vi "mxwScript_API_Option_TemplateRef.vi"(6 "terminalData":T2, 7 "templateRefType":T3, 8 "error in (no error)":errorcluster, 11 "options in":T4[](array[typedef])) -> (0 "error out":errorcluster, 3 "options out":T4[](array[typedef]))   [LabVIEW 2020]
doc: "Sets the default relationship between the template and block diagram reference points. This is used to calculate the drop position of templates."
uses:
  codeGenAPISupport.llb/cgAPI_mxwScript_OptionData.ctl
  codeGenAPISupport.llb/cgAPI_mxwScript_DrpTmplt_TemplateRefType.ctl
  codeGenAPISupport.llb/cgAPI_mxwScript_DrpTmplt_TerminalData.ctl
  codeGenAPISupport.llb/cgAPI_mxwScript_DrpTmplt_ReferencePosition.ctl
panel:
  in  "referencePosition":T1
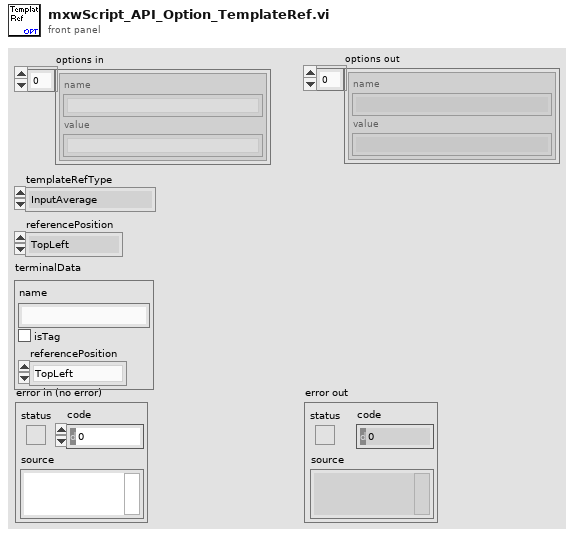
[diagram p1: front panel]
types:
  T1 = typedef "cgAPI_mxwScript_DrpTmplt_ReferencePosition.ctl" = enum16{"TopLeft", "Top", "TopRight", "Left", "Middle", "Right", "BottomLeft", "Bottom", "BottomRight"}
  T2 = typedef "cgAPI_mxwScript_DrpTmplt_TerminalData.ctl" = cluster{"name":string, "termIsTag":bool, "referencePosition":T1}
  T3 = typedef "cgAPI_mxwScript_DrpTmplt_TemplateRefType.ctl" = enum16{"InputAverage", "Absolute", "Terminal"}
  T4 = typedef "cgAPI_mxwScript_OptionData.ctl" = cluster{"name":string, "value":string}
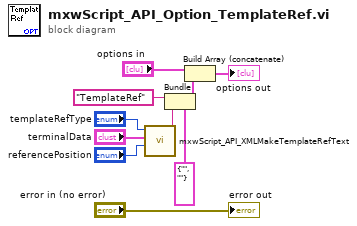
[diagram p0: block diagram]
diagram:
  n1 = call "mxwScript_API_XMLMakeTemplateRefText.vi"("referencePosition"="referencePosition", "terminalData"="terminalData", "templateRefType"="templateRefType") -> ("templateRefText"=w3:string)  [unwired: 8 out]
  n2 = Bundle(cluster=T4 {"name"="", "value"=""} ("optionData"), "name"="TemplateRef", "value"=w3) -> (w8:T4)
  n3 = Build Array (concatenate)("options in", w8) -> (→"options out":T4[])
  "error out" <- "error in (no error)"
